vi "test15-StateBroadcast_Event.vi"(8 "error in (no error)":errorcluster, 11 "TestCase in":refnum<class "testcase-CSMGlobalLog.lvclass">) -> (0 "error out":errorcluster, 3 "TestCase out":refnum<class "testcase-CSMGlobalLog.lvclass">)   [LabVIEW 2017, in "testcase-CSMGlobalLog.lvclass"]
uses:
  testcase-CSMGlobalLog.lvclass
  testcase-CSMGlobalLog.lvclass/testcase-CSMGlobalLog.ctl
  src/user.lib/_NEVSTOP/Communicable State Machine(CSM)/_Support/Typedef/_CSM_GlobalLog_MSG.ctl
  src/user.lib/_NEVSTOP/Communicable State Machine(CSM)/_Support/Typedef/_CSM_Response Source Message.ctl
  src/user.lib/_NEVSTOP/Communicable State Machine(CSM)/_Support/Typedef/_CSM_GlobalLog_MSG_TYPE.ctl
  127dd118-dd57-4e96-9fb1-428c5436480b.vi
  2d67c184-8a79-40d6-917b-f5673decc83c.vi
  c0dc643a-0362-49fc-99f4-5251266ba5a0.vi
  src/user.lib/_NEVSTOP/Communicable State Machine(CSM)/_Support/GlobalEvent/GEvt-Generate with Rule Check.vi
  src/user.lib/_NEVSTOP/Communicable State Machine(CSM)/AdvanceAPI/CSM - Convert Error to Argument.vi
  src/user.lib/_NEVSTOP/Communicable State Machine(CSM)/_Support/GlobalEvent/Cache-GEvt Refs.vi
  src/user.lib/_NEVSTOP/Communicable State Machine(CSM)/AdvanceAPI/CSM - Make String Arguments Safe.vi
  src/user.lib/_NEVSTOP/Communicable State Machine(CSM)/_Support/ChangeFlag/FlagInstance-GEvt Refs.vi
  src/user.lib/_NEVSTOP/Communicable State Machine(CSM)/AdvanceAPI/CSM - Keywords.vi
  src/user.lib/_NEVSTOP/Communicable State Machine(CSM)/_Support/ChangeFlag/ChangeFlag-Read.vi
  src/user.lib/_NEVSTOP/Communicable State Machine(CSM)/_Support/ChangeFlag/ChangeFlagDB.vi
  src/user.lib/_NEVSTOP/Communicable State Machine(CSM)/_Support/GlobalEvent/FGV-GlobalEventRef(lvlibp).vi
  src/user.lib/_NEVSTOP/Communicable State Machine(CSM)/_Support/GlobalEvent/FGV-GlobalEventQueues(lvlibp).vi
  src/user.lib/_NEVSTOP/Communicable State Machine(CSM)/_Support/GlobalEvent/GEvt-Valid Subscribers.vi
  src/user.lib/_NEVSTOP/Communicable State Machine(CSM)/_Support/GlobalEvent/LogFilter/LogFilter - Check.vi
  src/user.lib/_NEVSTOP/Communicable State Machine(CSM)/_Support/GlobalEvent/LogFilter/LogFilter.lvclass
  <vilib>/addons/_JKI Toolkits/VI Tester/TestCase.llb/TestCase.lvclass
  src/user.lib/_NEVSTOP/Communicable State Machine(CSM)/Communicable State Machine.lvlib
  C:/Program Files (x86)/National Instruments/LabVIEW 2017/vi.lib/addons/_JKI Toolkits/VI Tester/TestCase.llb/TestCase.lvclass
panel:
  out "String cache each loop":string
  out "LoopCount":i32
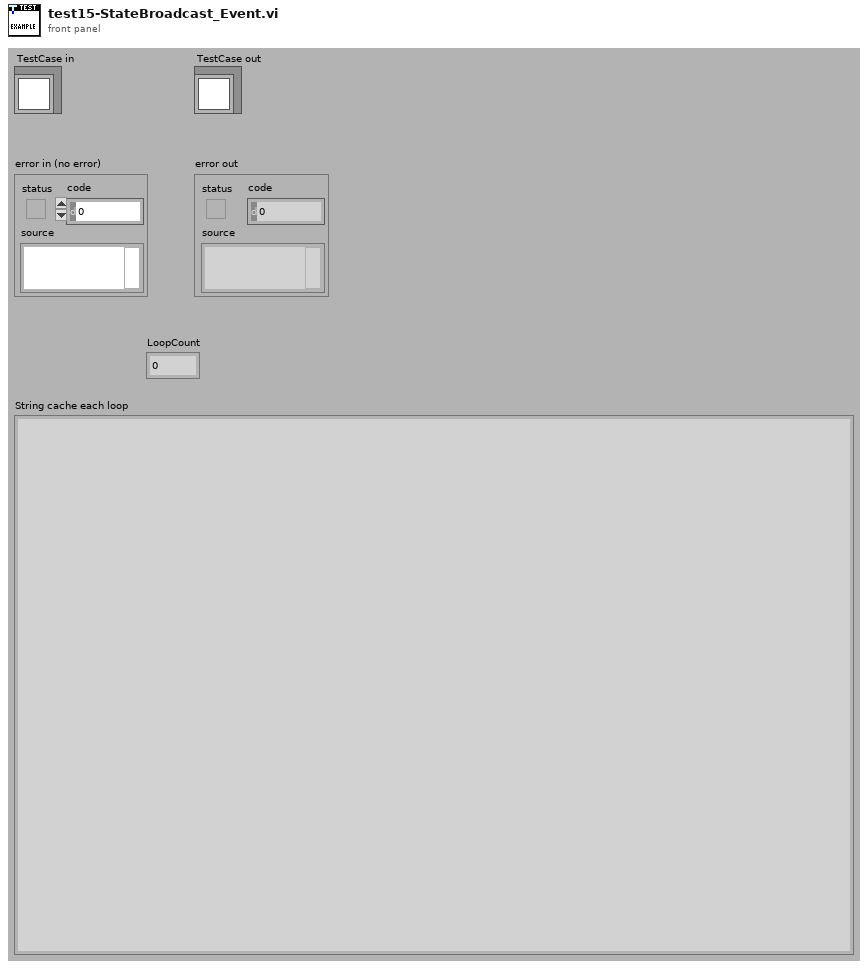
[diagram p1: front panel]
types:
  T1 = typedef "Communicable State Machine.lvlib/_CSM_GlobalLog_MSG.ctl" = cluster{"Name (\"\" to Use UUID)":string, "Current State":string, "Arguments":string, "Source Message":T2, "Source Module":string, "Complete(T)/Start(F)":bool, "LogType":T3, "Time Stamp":timestamp}
  T2 = typedef "Communicable State Machine.lvlib/_CSM_Response Source Message.ctl" = cluster{"‘State":string, "’Arguments":string, "’Error":errorcluster}
  T3 = typedef "Communicable State Machine.lvlib/_CSM_GlobalLog_MSG_TYPE.ctl" = enum16{"User Log", "State Change", "Status", "Interrupt", "Register", "Unregister", "Error Log", "Module Created", "Module Destroyed", "Async Message", "No-Rep Async Message", "Sync Message"}
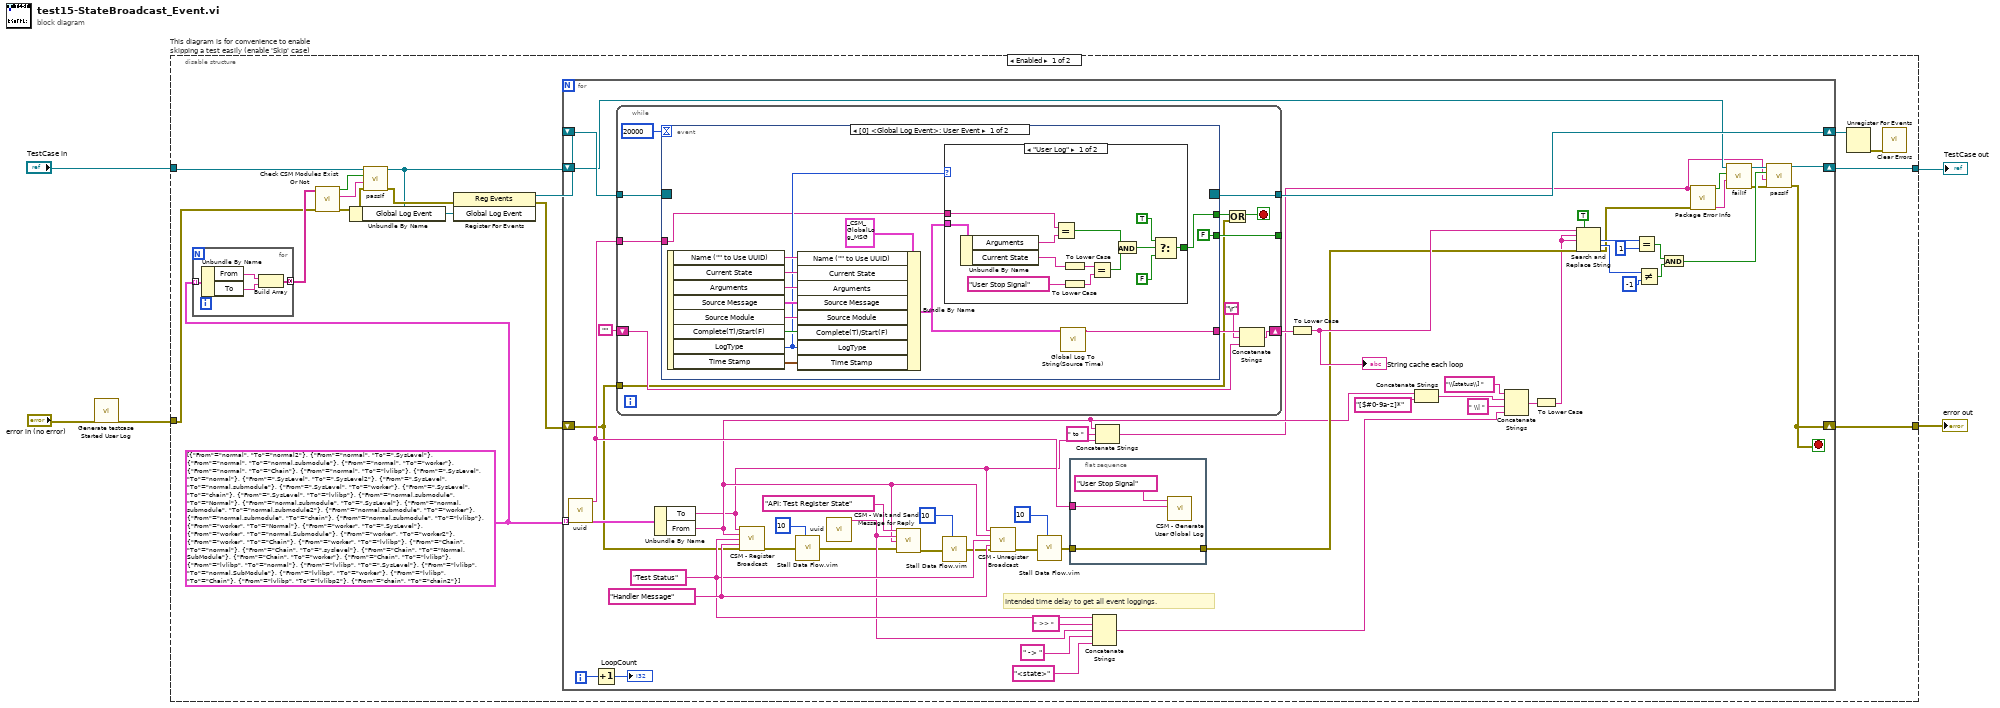
[diagram p0: block diagram]
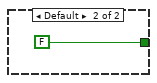
[diagram p2: hidden frame]
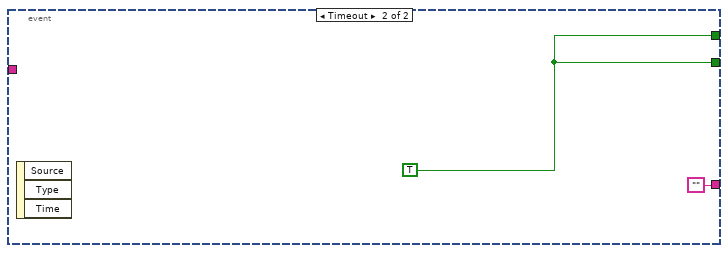
[diagram p3: hidden frame]
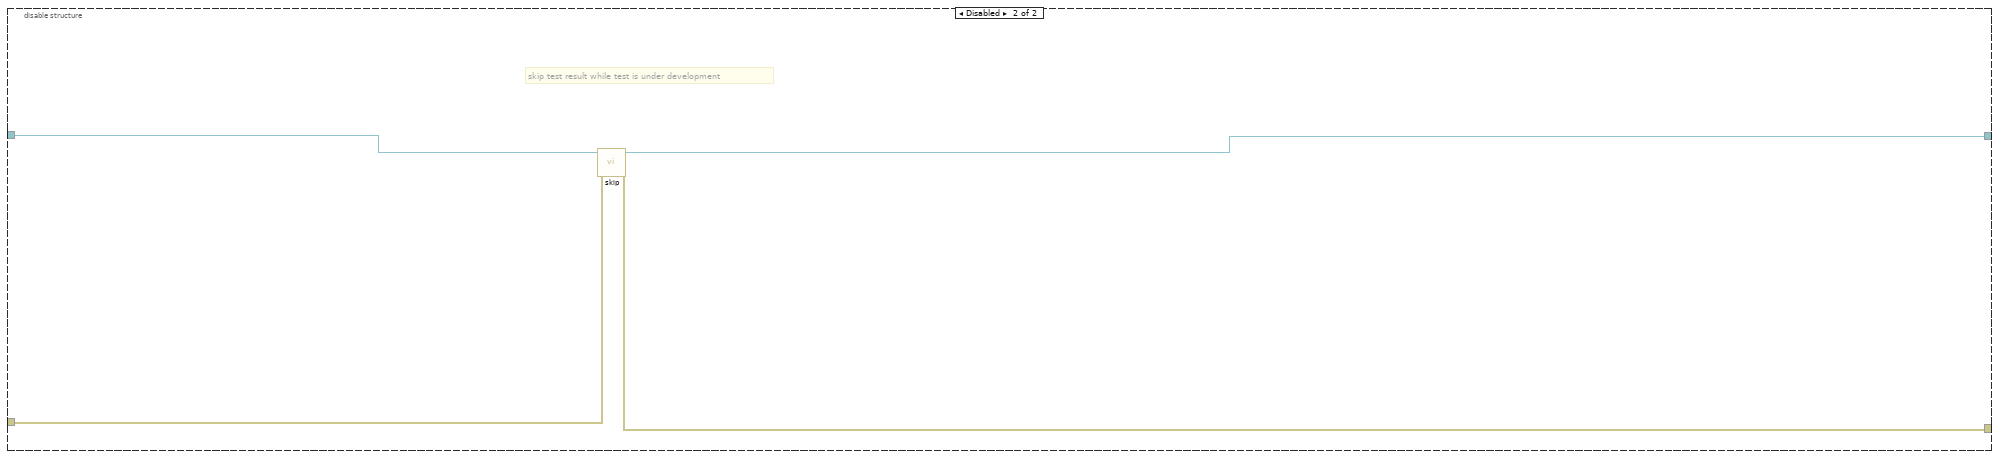
[diagram p4: hidden frame]
diagram:
  n1 = call "Generate testcase Started User Log.vi"("Error In"="error in (no error)") -> ("error out"=w1:errorcluster)  [unwired: 10 in]
  n2 = disable-structure "This diagram is for convenience to enable skipping a test easily (enable 'Skip' case)" shown="Enabled" {
    disable-tunnel: "TestCase in" -> [w11 w128]
    disable-tunnel: [w20 w126] -> w2
    disable-tunnel: [w19 w127] -> w4
    disable-tunnel: w1 -> [w9 w125]
    frame Enabled {
      w12 = cluster{"From":string, "To":string}[] [{"From"="normal", "To"="normal2"}, {"From"="normal", "To"=".SysLevel"}, {"From"="normal", "To"="normal.submodule"}, {"From"="normal", "To"="worker"}, {"From"="normal", "To"="Chain"}, {"From"="normal", "To"="lvlibp"}, {"From"=".SysLevel", "To"="normal"}, {"From"=".SysLevel", "To"=".SysLevel2"}, {"From"=".SysLevel", "To"="normal.submodule"}, {"From"=".SysLevel", "To"="worker"}, {"From"=".SysLevel", "To"="chain"}, {"From"=".SysLevel", "To"="lvlibp"}, {"From"="normal.submodule", "To"="Normal"}, {"From"="normal.submodule", "To"=".SysLevel"}, {"From"="normal.submodule", "To"="normal.submodule2"}, {"From"="normal.submodule", "To"="worker"}, {"From"="normal.submodule", "To"="chain"}, {"From"="normal.submodule", "To"="lvlibp"}, {"From"="worker", "To"="Normal"}, {"From"="worker", "To"=".SysLevel"}, {"From"="worker", "To"="normal.Submodule"}, {"From"="worker", "To"="worker2"}, {"From"="worker", "To"="Chain"}, {"From"="worker", "To"="lvlibp"}, {"From"="Chain", "To"="normal"}, {"From"="Chain", "To"=".syslevel"}, {"From"="Chain", "To"="Normal.SubModule"}, {"From"="Chain", "To"="worker"}, {"From"="Chain", "To"="lvlibp"}, {"From"="lvlibp", "To"="normal"}, {"From"="lvlibp", "To"=".SysLevel"}, {"From"="lvlibp", "To"="normal.SubModule"}, {"From"="lvlibp", "To"="worker"}, {"From"="lvlibp", "To"="Chain"}, {"From"="lvlibp", "To"="lvlibp2"}, {"From"="chain", "To"="chain2"}]
      n3 = for {
        tunnel: w12 -> [w25] mode=indexing
        tunnel: [w22] -> w16 mode=concatenating
        n4 = Unbundle By Name(w25) -> ("From"=w24:string, "To"=w23:string)
        n5 = Build Array(w24, w23) -> (w22:string[])
      }
      n6 = call "Check CSM Modules Exist Or Not.vi"("error in"=w9, "CSM names in"=w16) -> ("error out"=w14:errorcluster, "Debug string"=w15:string, "All Modules Exist?"=w17:bool)  [unwired: 7 in]
      n7 = call-dynamic "passIf.vi"("error in (no error)"=w14, "message (\"\")"=w15, "pass"=w17, "TestCase in"=w11) -> ("error out"=w13:errorcluster, "TestCase out"=w10:refnum<class "testcase-CSMGlobalLog.lvclass">)  [unwired: 6 in]
      n8 = Unbundle By Name(w10) -> ("Global Log Event"=w18:refnum<user-event>)
      n9 = register-events(error in=w13, w18) -> (reference out=w7:refnum<event-registration>, error out=w8:errorcluster)  [unwired: 1 in]
      n10 = for {
        shift-right: [w78] -> w21
        shift-left: w7 -> [w79]
        shift-right: [w75] -> w19
        shift-left: w8 -> [w32]
        tunnel: w12 -> [w56] mode=indexing
        shift-right: [w77] -> w20
        shift-left: w10 -> [w40]
        i -> [w64]
        stop <- w75 stop-if-true
        w59 = "Handler Message" ("API (If \"\", Same as Trigger)")
        w52 = "Test Status" ("Trigger")
        # "Intended time delay to get all event loggings."
        n11 = call "uuid.vi"() -> ("UUID"=w65:string)  [unwired: 11 in]
        n12 = Increment(x=w64) -> (x+1=→"LoopCount":i32)
        n13 = while {
          tunnel: w79 -> [w94]
          tunnel: [w93] -> w78
          shift-right: [w86] -> w60
          shift-left: "" -> [w89]
          tunnel: w65 -> [w91]
          tunnel: [w90] -> _
          tunnel: w32 -> [w83]
          stop <- w85 stop-if-true
          n14 = event shown="[0] <Global Log Event>: User Event" {
            selector: w94 -> [_ _]
            dyn-events: [_ _] -> w93
            timeout: 20000 -> [_ _]
            tunnel: [w95 ""] -> w88
            tunnel: [w97 w124] -> w84
            tunnel: w91 -> [w98 _]
            tunnel: [FALSE ("Stop") w124] -> w90
            event User Event {
              n15 = event-data() -> ("Name (\"\" to Use UUID)"=w107:string, "Current State"=w106:string, "Arguments"=w105:string, "Source Message"=w104:T2, "Source Module"=w103:string, "Complete(T)/Start(F)"=w102:bool, "LogType"=w99:T3, "Time Stamp"=w101:timestamp)  [unwired: 1 in]
              n16 = Bundle By Name(cluster=T1 {"Name (\"\" to Use UUID)"="", "Current State"="", "Arguments"="", "Source Message"={"‘State"="", "’Arguments"="", "’Error"={"status"=FALSE, "code"=0, "source"=""}}, "Source Module"="", "Complete(T)/Start(F)"=FALSE, "LogType"=enum."State Change", "Time Stamp"=timestamp(0 s since 1904-01-01)} ("Cross CSM Data"), "Name (\"\" to Use UUID)"=w107, "Current State"=w106, "Arguments"=w105, "Source Message"=w104, "Source Module"=w103, "Complete(T)/Start(F)"=w102, "LogType"=w99, "Time Stamp"=w101) -> (w96:T1)
              n17 = case shown="\"User Log\"" w99 {
                tunnel: w96 -> [w121 _]
                tunnel: w98 -> [w120 _]
                tunnel: [w109 FALSE] -> w97
                frame "User Log" {
                  n18 = Unbundle By Name(w121) -> ("Arguments"=w119:string, "Current State"=w118:string)
                  n19 = Equal?(x=w120, y=w119) -> (x = y?=w113:bool)
                  n20 = To Lower Case(string=w118) -> (all lower case string=w117:string)
                  n21 = To Lower Case(string="User Stop Signal" ("Log")) -> (all lower case string=w115:string)
                  n22 = Equal?(x=w117, y=w115) -> (x = y?=w114:bool)
                  n23 = And(x=w113, y=w114) -> (x .and. y?=w112:bool)
                  n24 = Select(t=TRUE, s=w112, f=FALSE) -> (s? t:f=w109:bool)
                }
                frame Default {
                }
              }
              n25 = call "Global Log To String(Source Time).vi"("Log"=w96) -> ("Log String"=w95:string)  [unwired: 9 in]
            }
            event Timeout {
              w124 = TRUE ("Stop")
              n26 = event-data() -> ()  [unwired: 1 in, 3 out]
            }
          }
          n27 = Or(x=w84, y=w83) -> (x .or. y?=w85:bool)
          n28 = Concatenate Strings(w88, "\r", w89) -> (w86:string)
        }
        n29 = Unbundle By Name(w56) -> ("To"=w35:string, "From"=w36:string)
        n30 = call "CSM - Register Broadcast.vi"("CSM Name(Empty for Broadcast Event)"=w35, "Source CSM Name (* as Default)"=w36, "Trigger"=w52, "API (If \"\", Same as Trigger)"=w59, "Error In"=w32) -> ("error out"=w27:errorcluster)  [unwired: 9 in, 1 out]
        n31 = call "Stall Data Flow.vim"("value in"=w27, "milliseconds to wait"=u32 10) -> ("value out"=w26:errorcluster)  [unwired: 1 out]
        n32 = call "uuid.vi"() -> ("UUID"=w51:string)  [unwired: 11 in]
        n33 = call "CSM - Wait and Send Message for Reply.vi"("State"="API: Test Register State", "Arguments (\"\")"=w51, "Target Module"=w36, "Error In (No Error)"=w26) -> ("error out"=w30:errorcluster)  [unwired: 8 in, 3 out]
        n34 = call "Stall Data Flow.vim"("value in"=w30, "milliseconds to wait"=u32 10) -> ("value out"=w29:errorcluster)  [unwired: 1 out]
        n35 = call "CSM - Unregister Broadcast.vi"("CSM Name(Empty for Broadcast Event)"=w35, "Source CSM Name (* as Default)"=w36, "Trigger"=w52, "API (\"*\" as Default)"=w59, "Error In"=w29) -> ("error out"=w57:errorcluster)  [unwired: 9 in, 1 out]
        n36 = call "Stall Data Flow.vim"("value in"=w57, "milliseconds to wait"=u32 10) -> ("value out"=w66:errorcluster)  [unwired: 1 out]
        n37 = flat-sequence {
          tunnel: w65 -> [w81]
          tunnel: w66 -> [w80]
          tunnel: [w80] -> w61
          frame #0 {
            n38 = call "CSM - Generate User Global Log.vi"("Arguments"=w81, "Log"="User Stop Signal") -> ()  [unwired: 9 in, 1 out]
          }
        }
        n39 = Concatenate Strings(w52, " >> " ("string"), w51, " -> " ("string"), "<state>" ("search string")) -> (w44:string)
        n40 = Concatenate Strings(w36, " to " ("string"), w35) -> (w33:string)
        n41 = To Lower Case(string=w60) -> (all lower case string=w62:string)
        "String cache each loop" <- w62
        n42 = Concatenate Strings(w36, "[$#0-9a-z]*" ("string")) -> (w45:string)
        n43 = Concatenate Strings("\\[status\\] " ("regular expression"), w45, " \\| " ("string"), w44) -> (w48:string)
        n44 = To Lower Case(string=w48) -> (all lower case string=w43:string)
        n45 = Search and Replace String(replace all?=TRUE ("replace all? (F)"), input string=w62, search string=w43, replace string=w43, error in=w61) -> (number of replacements=w71:i32, offset past replacement=w72:i32, error out=w37:errorcluster)  [unwired: 3 in, 1 out]
        n46 = Equal?(x=w71, y=1) -> (x = y?=w73:bool)
        n47 = Not Equal?(x=w72, y=-1) -> (x != y?=w74:bool)
        n48 = And(x=w73, y=w74) -> (x .and. y?=w50:bool)
        n49 = call "Package Error Info.vi"("error in"=w37, "String in"=w33) -> ("packed error info out"=w41:string, "error status"=w42:bool)  [unwired: 8 in]
        n50 = call-dynamic "failIf.vi"("message (\"\")"=w41, "fail"=w42, "TestCase in"=w40) -> ("error out"=w38:errorcluster, "TestCase out"=w39:refnum<class "testcase-CSMGlobalLog.lvclass">)  [unwired: 7 in]
        n51 = call-dynamic "passIf.vi"("error in (no error)"=w38, "message (\"\")"=w33, "pass"=w50, "TestCase in"=w39) -> ("error out"=w75:errorcluster, "TestCase out"=w77:refnum<class "testcase-CSMGlobalLog.lvclass">)  [unwired: 6 in]
      }
      n52 = Unregister For Events(event registration refnum=w21) -> (error out=w6:errorcluster)  [unwired: 1 in]
      n53 = call <vilib>:"Clear Errors.vi"("error in (no error)"=w6) -> ()  [unwired: 5 in, 2 out]
    }
    frame Disabled {
      # "skip test result while test is under development"
      n54 = call <vilib>:"skip.vi"("error in (no error)"=w125, "TestCase in"=w128) -> ("error out"=w127:errorcluster, "TestCase out"=w126:refnum<class "testcase-CSMGlobalLog.lvclass">)  [unwired: 8 in]
    }
  }
  "error out" <- w4
  "TestCase out" <- w2
